vi "Webcam simply example.vi"(8 "error in (no error)":errorcluster) -> (0 "error out":errorcluster)   [LabVIEW 2012]
doc: "VI for streaming video from a webcam and show the temperature.\nBased on LibVLC.dll (http://www.videolan.org/) , needs an installation of this software to run.\nThe portable version of VLC is attached to the project"
uses:
  Controls-Webcam/VLC Var.ctl
  SubVIs-Webcam/subs/StartVideo PictureBox.vi
  System.Windows.Forms
panel:
  in  "PictureBox":refnum<k24>(container)
  in  "Exit":bool
  # "C:\\Program Files (x86)\\VideoLAN\\VLC\\libvlc.dll"
  # "C:\\Archivos de programa\\VideoLAN\\VLC\\libvlc.dll"
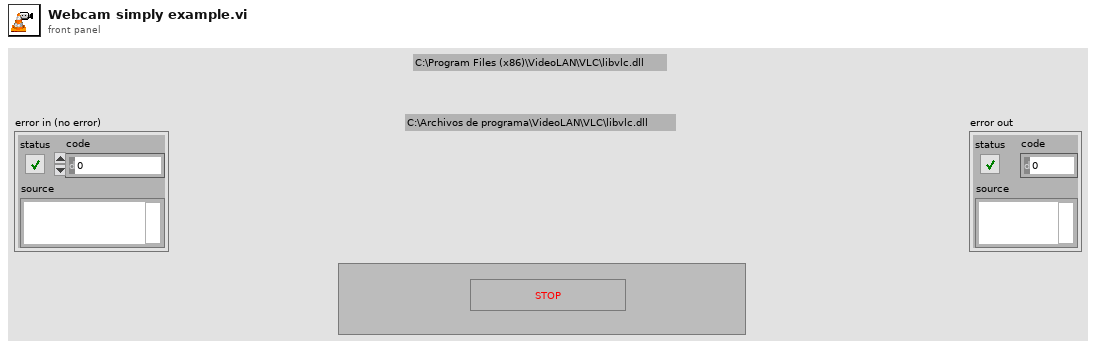
[diagram p1: front panel]
types:
  T1 = typedef "VLC Var.ctl" = cluster{"DLL Path":path, "p_i":i32, "p_md":i32, "p_mi":i32, "Player State":i32, "VLC Process Ref":refnum<k24>, "Drawable":i32}
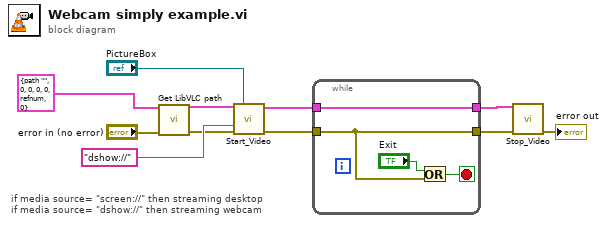
[diagram p0: block diagram]
diagram:
  # "if media source= \"screen://\" then streaming desktop\nif media source= \"dshow://\" then streaming webcam"
  n1 = call "Get LibVLC path.vi"("VLC Variables In"=T1 {"DLL Path"=path "", "p_i"=0, "p_md"=0, "p_mi"=0, "Player State"=0, "VLC Process Ref"=refnum, "Drawable"=0}, "error in (no error)"="error in (no error)") -> ("VLC Variables Out"=w3:T1, "error out"=w7:errorcluster)  [unwired: 12 in]
  n2 = call-poly "Start_Video.vi"("VLC Variables In"=w3, "PictureBox"="PictureBox", "Media Source"="dshow://", "error in (no error)"=w7) -> ("VLC Variables Out"=w9:T1, "error out"=w2:errorcluster)  [unwired: 10 in]
  n3 = while {
    tunnel: w9 -> [w13]
    tunnel: [w13] -> w5
    tunnel: [w12] -> w4
    tunnel: w2 -> [w12]
    stop <- w15 stop-if-true
    n4 = Or(x="Exit", y=w12) -> (x .or. y?=w15:bool)
  }
  n5 = call "Stop_Video.vi"("VLC Variables In"=w5, "error in (no error)"=w4) -> ("error out"=→"error out":errorcluster)  [unwired: 13 in]
